vi "Arduino.vi"(1 "Encender":bool, 2 "VISA resource":refnum<visa-resource-name>) -> (0 "Boolean":bool)   [LabVIEW 2011]
uses:
  <vilib>/LabVIEW Interface for Arduino/LabVIEW Interface for Arduino.lvlib
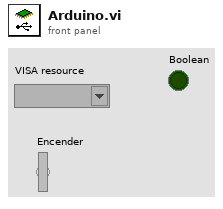
[diagram p1: front panel]
types:
  T1 = typedef "LabVIEW Interface for Arduino.lvlib/Arduino Resource.ctl" = cluster{"VISA resource":refnum<visa-resource-name>, "Board Type":T2, "Connection Type":enum8{"USB / Serial"}, "Bytes Per Packet (15)":u8}
  T2 = typedef "LabVIEW Interface for Arduino.lvlib/Board Type.ctl" = enum16{"Uno", "Mega 2560"}
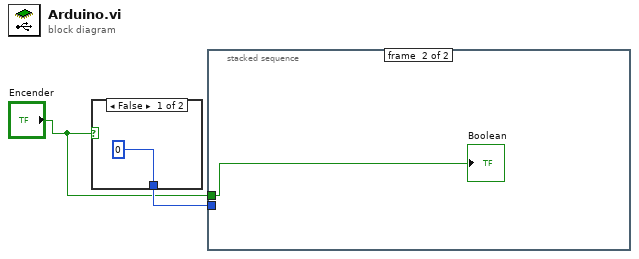
[diagram p0: block diagram]
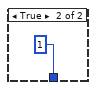
[diagram p2: hidden frame]
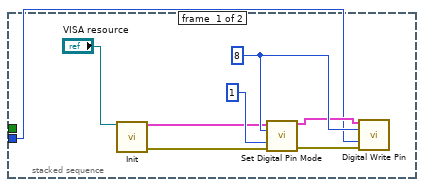
[diagram p3: hidden frame]
diagram:
  n1 = case shown="False" "Encender" {
    tunnel: [0 1] -> w2
    frame False {
    }
    frame True {
    }
  }
  n2 = stacked-sequence {
    tunnel: w2 -> [w5 _]
    tunnel: "Encender" -> [_ w13]
    frame #0 {
      w12 = 8
      n3 = call <vilib>:"Init.vi"("VISA resource"="VISA resource") -> ("Arduino Resource"=w10:T1, "error out"=w9:errorcluster)  [unwired: 17 in]
      n4 = call <vilib>:"Set Digital Pin Mode.vi"("Arduino Resource"=w10, "Digital I/O Pin"=w12, "Pin Mode (Input)"=1, "error in"=w9) -> ("Arduino Resource"=w7:T1, "error out"=w8:errorcluster)  [unwired: 10 in]
      n5 = call <vilib>:"Digital Write Pin.vi"("Arduino Resource"=w7, "Digital I/O Pin (0)"=w12, "Value (0)"=w5, "error in"=w8) -> ()  [unwired: 10 in, 2 out]
    }
    frame #1 {
      "Boolean" <- w13
    }
  }
